vi "nand-3-input.vi"(8 "z":bool, 10 "y":bool, 11 "x":bool) -> (1 "NAND":bool)   [LabVIEW 2021]
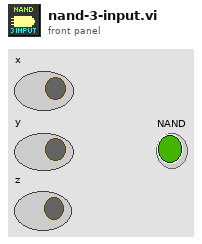
[diagram p1: front panel]
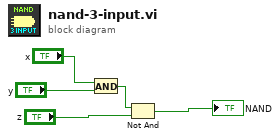
[diagram p0: block diagram]
diagram:
  n1 = And(x="x", y="y") -> (x .and. y?=w5:bool)
  n2 = Not And(1:"z", 2:w5) -> (0:→"NAND":bool)
